vi "Subset Buffer.vi"(8 "error in (no error)":errorcluster, 9 "size":u64 format="%d bytes", 10 "offset":u64 format="%d bytes", 11 "Buffer in":refnum<class "Buffer.lvclass">) -> (0 "error out":errorcluster, 1 "offset + size":u64 format="%d bytes", 2 "subset Buffer":refnum<class "Buffer.lvclass">, 3 "Buffer out":refnum<class "Buffer.lvclass">)   [LabVIEW 2017, in "DSF Core.lvlib" / "Buffer.lvclass"]
doc: "Creates a new <b>subset Buffer</b> that encapsulates a subset of <b>Buffer</b> that is <b>size</b> bytes in length, and located at <b>offset</b> bytes.\n\nThe <b>subset Buffer</b> must be within the bounds of <b>Buffer</b>."
uses:
  Buffer.lvclass
  C:/Git/DSF/LabVIEW-Memory/Source/Classes/Pointer/Pointer.lvclass
  Buffer.lvclass/Buffer.ctl
  LabVIEW-Memory/Source/Classes/Pointer/Pointer.lvclass
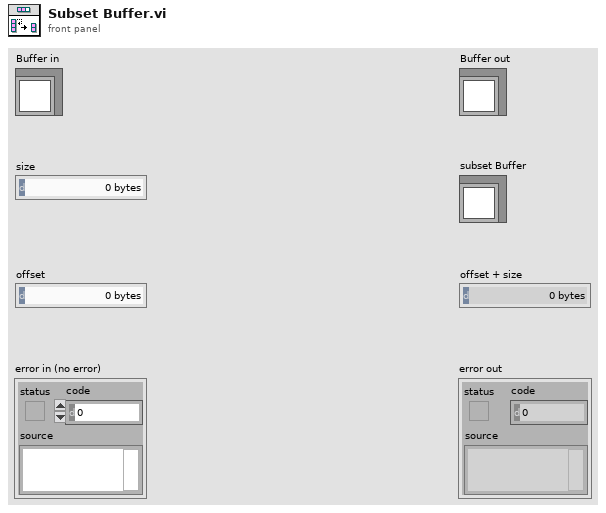
[diagram p1: front panel]
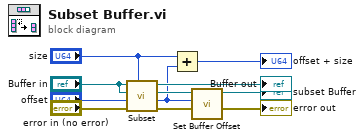
[diagram p0: block diagram]
diagram:
  n1 = call "Subset.vi"("length (-1: rest)"="size", "error in (no error)"="error in (no error)", "offset (0)"="offset", "subset Pointer type"="Buffer in", "base Pointer in"="Buffer in") -> ("error out"=→"error out":errorcluster, "offset out"=w2:u64, "subset Pointer"=w3:refnum<class "Buffer.lvclass">, "base Pointer out"=→"Buffer out":refnum<class "Buffer.lvclass">)  [unwired: 3 in]
  n2 = Add(x="size", y=w2) -> (x+y=→"offset + size":u64)
  n3 = call "Set Buffer Offset.vi"("buffer offset"=w2, "Buffer in"=w3) -> ("Buffer out"=→"subset Buffer":refnum<class "Buffer.lvclass">)  [unwired: 9 in]
